vi "Custom Device Template Tool.vi"(4 "Extra Page Names (No Extension)":string[](array[string]), 6 "Open Project":bool=TRUE, 7 "Overwrite Existing (T)":bool=TRUE, 8 "error in (no error)":errorcluster, 9 "Execution Mode":T1, 10 "Custom Device Name (No Extension)":string, 11 "Target Folder":path=path "c:/temp") -> (0 "error out":errorcluster, 1 "Custom Device Library path":path, 2 "Custom Device Project path":path)   [LabVIEW 2020, in "Custom Device Template Tool.lvlib"]
uses:
  <vilib>/NI VeriStand/Custom Device Tools/Custom Device Template Tool/Custom Device Template Tool.lvlib
  <vilib>/NI VeriStand/Custom Device API/Custom Device Execution Mode.ctl
  NationalInstruments.VeriStand.Internal
  <vilib>/NI VeriStand/Custom Device API/Initialization VI Template.vit
  <vilib>/NI VeriStand/Custom Device API/Page Template.vit
  <vilib>/NI VeriStand/Custom Device API/Inline Custom Device Driver VI Template (HW Interface).vit
  <vilib>/NI VeriStand/Custom Device API/Inline Custom Device Driver VI Template (Model Interface).vit
  <vilib>/NI VeriStand/Custom Device API/Custom Device API.lvlib
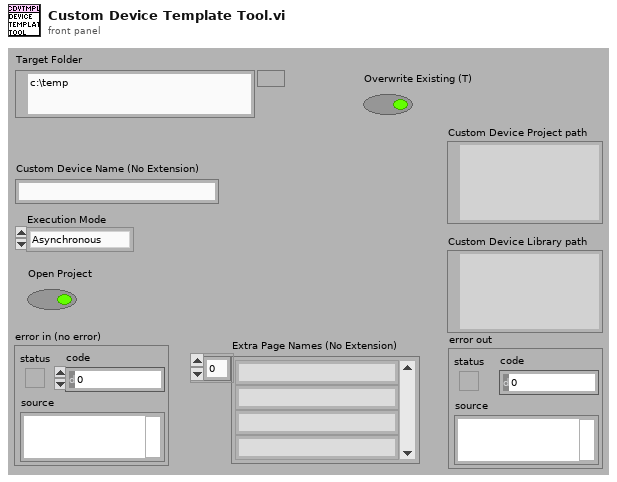
[diagram p1: front panel]
types:
  T1 = typedef "Custom Device API.lvlib/Custom Device Execution Mode.ctl" = enum16{"Asynchronous", "Inline HW Interface", "Inline Model Interface", "Inline Timing and Sync", "Asynchronous Timing and Sync"}
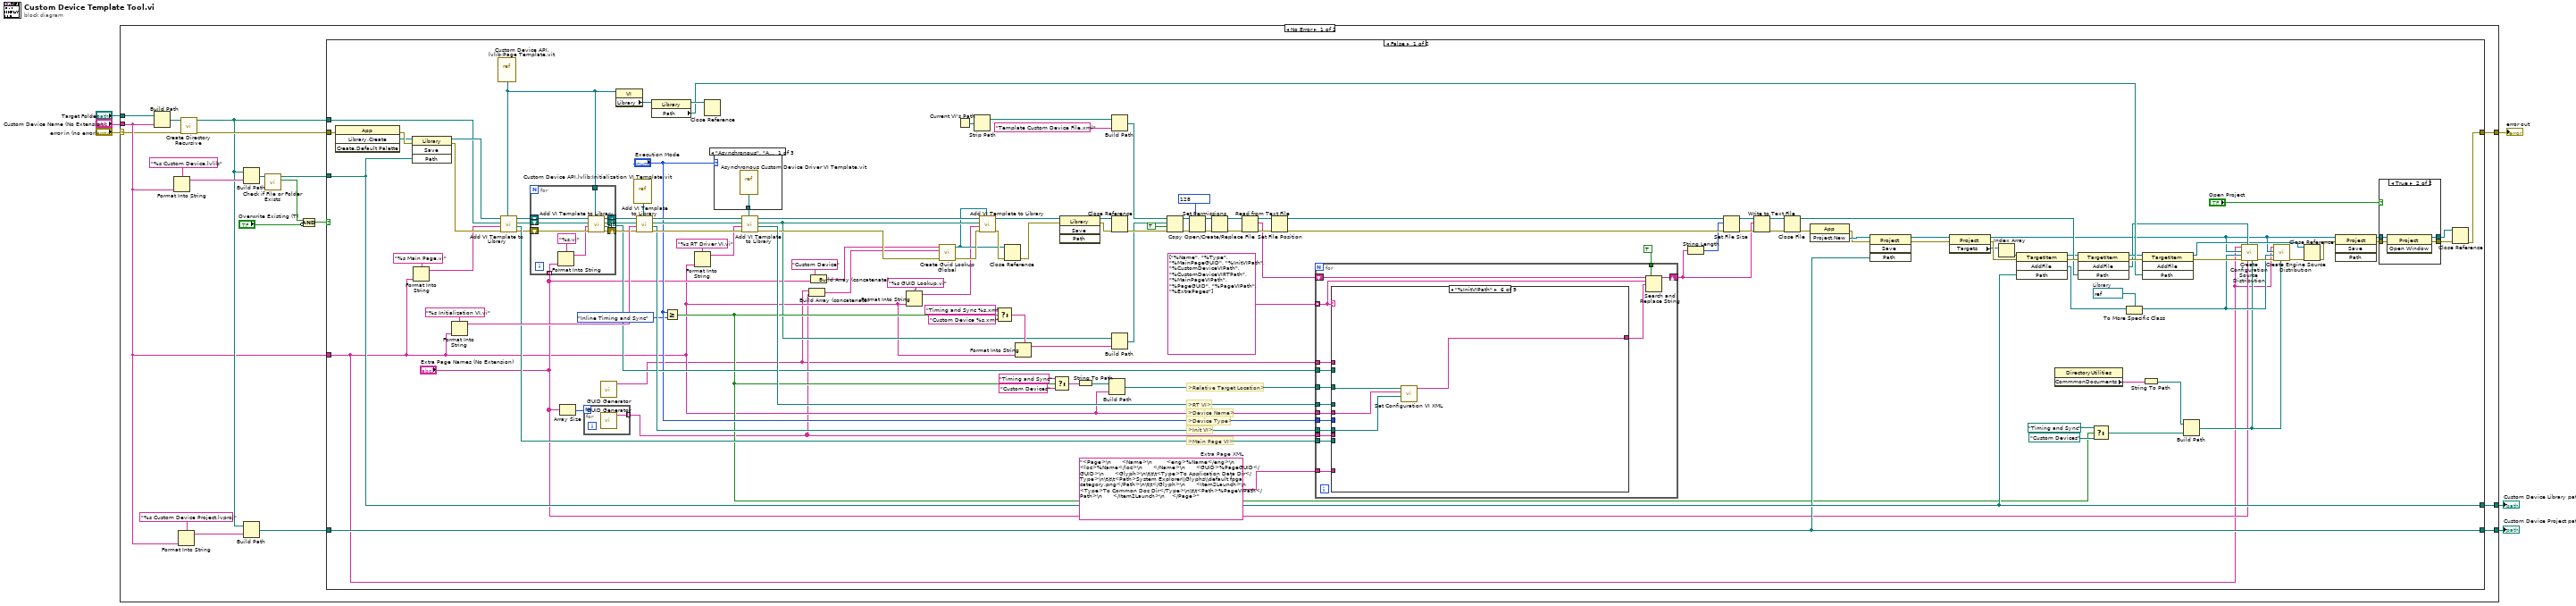
[diagram p0: block diagram]
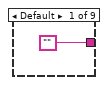
[diagram p3: hidden frame]
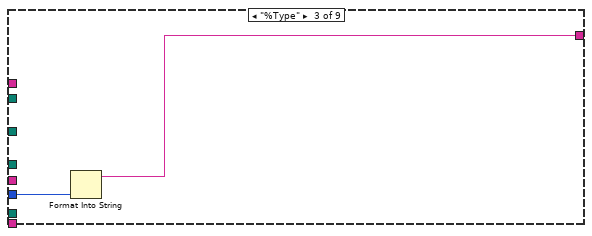
[diagram p5: hidden frame]
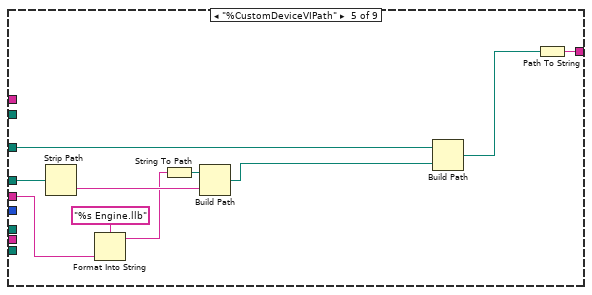
[diagram p7: hidden frame]
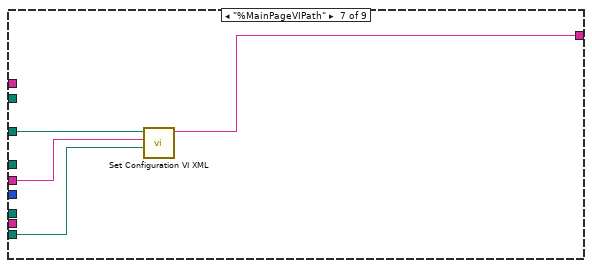
[diagram p8: hidden frame]
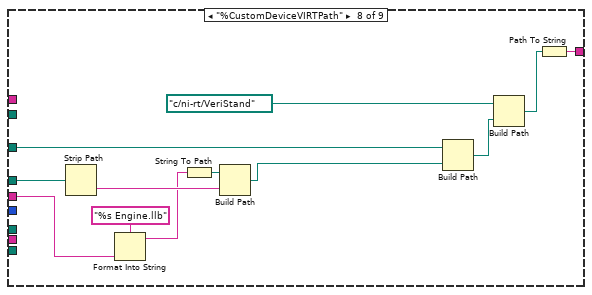
[diagram p9: hidden frame]
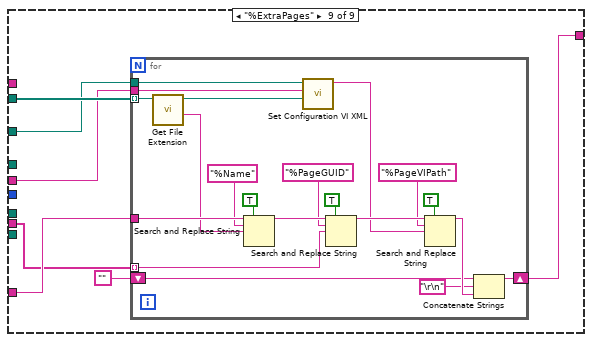
[diagram p10: hidden frame]
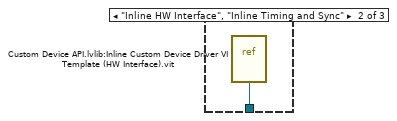
[diagram p11: hidden frame]
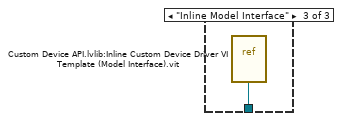
[diagram p12: hidden frame]
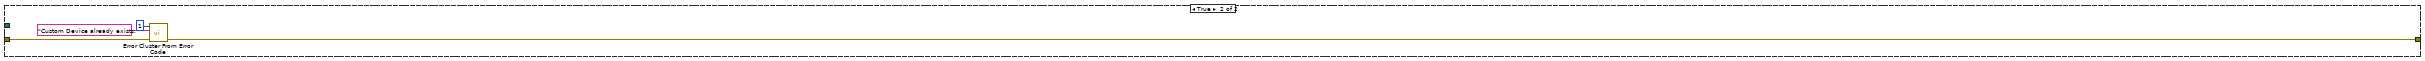
[diagram p13: hidden frame]
diagram:
  n1 = case shown="No Error" "error in (no error)" {
    selector: "error in (no error)" -> [w9 w256]
    tunnel: "Target Folder" -> [w21 _]
    tunnel: [w20 w256] -> w5
    tunnel: "Custom Device Name (No Extension)" -> [w16 _]
    tunnel: [w8 _] -> w2
    tunnel: [w7 _] -> w1
    frame No Error {
      n2 = Build Path(base path=w21, name or relative path=w16) -> (appended path=w25:path)
      n3 = Format Into String(format string="%s Custom Device.lvlib", w16) -> (resulting string=w22:string)  [unwired: 2 in, 1 out]
      n4 = Format Into String(format string="%s Custom Device Project.lvproj", w16) -> (resulting string=w19:string)  [unwired: 2 in, 1 out]
      n5 = call <vilib>:"Create Directory Recursive.vi"("error in (no error)"=w9, "directory"=w25) -> ("error out"=w23:errorcluster, "directory copy"=w17:path)  [unwired: 1 in, 3 out]
      n6 = Build Path(base path=w17, name or relative path=w22) -> (appended path=w14:path)
      n7 = Build Path(base path=w17, name or relative path=w19) -> (appended path=w15:path)
      n8 = call <vilib>:"Check if File or Folder Exists.vi"("path"=w14) -> ("file or folder exists?"=w12:bool, "dup path"=w13:path)  [unwired: 1 in, 8 out]
      n9 = Compound Arithmetic op=AND(w12, invert "Overwrite Existing (T)") -> (w10:bool)
      n10 = case shown="False" w10 {
        tunnel: w23 -> [w145 w255]
        tunnel: [w93 w254] -> w20
        tunnel: w17 -> [w84 _]
        tunnel: w16 -> [w31 _]
        tunnel: w15 -> [w57 _]
        tunnel: w13 -> [w58 _]
        tunnel: [w58 _] -> w8
        tunnel: [w57 _] -> w7
        frame False {
          w59 = "<Page>\n      <Name>\n        <eng>%Name</eng>\n        <loc>%Name</loc>\n      </Name>\n      <GUID>%PageGUID</GUID>\n      <Glyph>\n\t\t\t<Type>To Application Data Dir</Type>\n\t\t\t<Path>System Explorer\\Glyphs\\default fpga category.png</Path>\n\t\t</Glyph>\n      <Item2Launch>\n        <Type>To Common Doc Dir</Type>\n\t\t<Path>%PageVIPath</Path>\n      </Item2Launch>\n    </Page>"  # Extra Page XML
          w78 = refnum<vi> refnum  # Library
          # ">Relative Target Location>"
          # ">Device Type>"
          # ">Main Page VI>"
          # ">RT VI>"
          # ">Device Name>"
          # ">Init VI>"
          n11 = invoke class="App" method="Library.Create"(error in=w145) -> (error out=w147:errorcluster, "Create Library"=w146:refnum<vi>)  [unwired: 3 in, 2 out]
          n12 = invoke class="Library" method="Save"(reference=w146, error in=w147, "Path"=w58) -> (reference out=w143:refnum<vi>, error out=w148:errorcluster)  [unwired: 1 in, 2 out]
          n13 = Format Into String(format string="%s Main Page.vi", w31) -> (resulting string=w142:string)  [unwired: 2 in, 1 out]
          n14 = Format Into String(format string="%s Initialization VI.vi", w31) -> (resulting string=w139:string)  [unwired: 2 in, 1 out]
          n15 = vi-ref "Custom Device API.lvlib:Page Template.vit"() -> (w61:refnum<vi>)
          n16 = call <vilib>:"Add VI Template to Library.vi"("Template VI Refnum"=w61, "error in"=w148, "VI Name"=w142, "Custom Device Folder"=w84, "Custom Device Library in"=w143) -> ("error out"=w63:errorcluster, "VI Path out"=w117:path, "Custom Device Folder out"=w65:path, "Custom Device Library out"=w67:refnum<vi>)  [unwired: 3 out]
          n17 = for {
            shift-right: [w161] -> w66
            shift-left: w67 -> [w164]
            shift-right: [w160] -> w64
            shift-left: w65 -> [w163]
            shift-right: [w159] -> w62
            shift-left: w63 -> [w162]
            tunnel: w61 -> [w165]
            tunnel: "Extra Page Names (No Extension)" -> [w157] mode=indexing
            tunnel: [w155] -> w60 mode=indexing
            n18 = Format Into String(format string="%s.vi", w157) -> (resulting string=w156:string)  [unwired: 2 in, 1 out]
            n19 = call <vilib>:"Add VI Template to Library.vi"("Template VI Refnum"=w165, "error in"=w162, "VI Name"=w156, "Custom Device Folder"=w163, "Custom Device Library in"=w164) -> ("error out"=w159:errorcluster, "VI Path out"=w155:path, "Custom Device Folder out"=w160:path, "Custom Device Library out"=w161:refnum<vi>)  [unwired: 3 out]
          }
          n20 = Array Size(array="Extra Page Names (No Extension)") -> (size(s)=w43:i32)
          n21 = for {
            N: w43 -> [_]
            tunnel: [w154] -> w30 mode=indexing
            n22 = call <vilib>:"GUID Generator.vi"() -> ("GUID"=w154:string)  [unwired: 11 out]
          }
          n23 = call <vilib>:"GUID Generator.vi"() -> ("GUID"=w28:string)  [unwired: 11 out]
          n24 = property class="VI"(reference=w61) -> ("Library"=w92:refnum<vi>)  [unwired: 1 in, 2 out]
          n25 = vi-ref "Custom Device API.lvlib:Initialization VI Template.vit"() -> (w140:refnum<vi>)
          n26 = call <vilib>:"Add VI Template to Library.vi"("Template VI Refnum"=w140, "error in"=w62, "VI Name"=w139, "Custom Device Folder"=w64, "Custom Device Library in"=w66) -> ("error out"=w149:errorcluster, "VI Path out"=w116:path, "Custom Device Folder out"=w134:path, "Custom Device Library out"=w135:refnum<vi>)  [unwired: 3 out]
          n27 = property class="Library"(reference=w92) -> (reference out=w91:refnum<vi>, "Path"=w89:path)  [unwired: 1 in, 1 out]
          n28 = Greater Or Equal?(x="Execution Mode", y=Custom_Device_Execution_Mode."Inline Timing and Sync") -> (x >= y?=w47:bool)
          n29 = Format Into String(format string="%s RT Driver VI.vi", w31) -> (resulting string=w138:string)  [unwired: 2 in, 1 out]
          n30 = Close Reference(reference=w91) -> ()  [unwired: 1 in, 1 out]
          n31 = case shown="\"Asynchronous\", \"Asynchronous Timing and Sync\"" "Execution Mode" {
            tunnel: [w249 w250 w251] -> w137
            frame "Asynchronous", "Asynchronous Timing and Sync" {
              n32 = vi-ref <vilib>:"Asynchronous Custom Device Driver VI Template.vit"() -> (w249:refnum<vi>)
            }
            frame "Inline HW Interface", "Inline Timing and Sync" {
              n33 = vi-ref "Custom Device API.lvlib:Inline Custom Device Driver VI Template (HW Interface).vit"() -> (w250:refnum<vi>)
            }
            frame "Inline Model Interface" {
              n34 = vi-ref "Custom Device API.lvlib:Inline Custom Device Driver VI Template (Model Interface).vit"() -> (w251:refnum<vi>)
            }
          }
          n35 = call <vilib>:"Add VI Template to Library.vi"("Template VI Refnum"=w137, "error in"=w149, "VI Name"=w138, "Custom Device Folder"=w134, "Custom Device Library in"=w135) -> ("error out"=w40:errorcluster, "VI Path out"=w150:path, "Custom Device Folder out"=w38:path, "Custom Device Library out"=w41:refnum<vi>)  [unwired: 3 out]
          n36 = Build Array (concatenate)(w28, w30) -> (w29:string[])
          n37 = Build Array (concatenate)("Custom Device", "Extra Page Names (No Extension)") -> (w32:string[])
          n38 = Format Into String(format string="%s GUID Lookup.vi", w31) -> (resulting string=w35:string)  [unwired: 2 in, 1 out]
          n39 = call <vilib>:"Create Guid Lookup Global.vi"("error in (no error)"=w40, "GUIDs"=w29, "Page Names"=w32) -> ("error out"=w39:errorcluster, "Global VI Refnum"=w36:refnum<vi>)  [unwired: 7 in]
          n40 = Current VI's Path() -> (path=w83:path)
          n41 = Strip Path(path=w83) -> (stripped path=w82:path)  [unwired: 1 out]
          n42 = call <vilib>:"Add VI Template to Library.vi"("Template VI Refnum"=w36, "error in"=w39, "VI Name"=w35, "Custom Device Folder"=w38, "Custom Device Library in"=w41) -> ("error out"=w153:errorcluster, "Custom Device Library out"=w42:refnum<vi>)  [unwired: 5 out]
          n43 = Select(t="Timing and Sync %s.xml" ("format string"), s=w47, f="Custom Device %s.xml" ("format string")) -> (s? t:f=w52:string)
          n44 = Close Reference(reference=w36, error in (no error)=w153) -> (error out=w152:errorcluster)
          n45 = Format Into String(format string=w52, w31) -> (resulting string=w131:string)  [unwired: 2 in, 1 out]
          n46 = Select(t="Timing and Sync", s=w47, f="Custom Devices" ("name or relative path")) -> (s? t:f=w44:string)
          n47 = invoke class="Library" method="Save"(reference=w42, error in=w152) -> (reference out=w100:refnum<vi>, error out=w99:errorcluster)  [unwired: 2 in, 2 out]
          n48 = String To Path(string=w44) -> (path=w115:path)
          n49 = Build Path(base path=w115, name or relative path=w31) -> (appended path=w114:path)
          n50 = Build Path(base path=w82, name or relative path="Template Custom Device File.xml") -> (appended path=w132:path)
          n51 = Close Reference(reference=w100, error in (no error)=w99) -> (error out=w133:errorcluster)
          n52 = Build Path(base path=w38, name or relative path=w131) -> (appended path=w130:path)
          n53 = Copy(8:w133, 9:TRUE ("overwrite (F)"), 10:w130, 11:w132) -> (0:w127:errorcluster, 3:w128:path)  [unwired: 2 out]
          n54 = Set Permissions(7:i16 128 ("permissions"), 8:w127, 11:w128) -> (0:w125:errorcluster, 3:w126:path)  [unwired: 2 out]
          n55 = Open/Create/Replace File(file path (use dialog)=w126, error in=w125) -> (refnum out=w124:refnum<file>, error out=w123:errorcluster)  [unwired: 5 out]
          n56 = Read from Text File(file (use dialog)=w124, error in=w123) -> (refnum out=w122:refnum<file>, text=w119:string, error out=w121:errorcluster)  [unwired: 3 out]
          n57 = Set File Position(refnum=w122, error in=w121) -> (refnum out=w113:refnum<file>, error out=w112:errorcluster)  [unwired: 2 out]
          n58 = for {
            tunnel: string[] ["%Name", "%Type", "%MainPageGUID", "%InitVIPath", "%CustomDeviceVIPath", "%CustomDeviceVIRTPath", "%MainPageVIPath", "%PageGUID", "%PageVIPath", "%ExtraPages"] ("array") -> [w182] mode=indexing
            shift-right: [w176] -> w108
            shift-left: w119 -> [w186]
            tunnel: TRUE ("replace all? (F)") -> [w185]
            tunnel: w31 -> [w184]
            tunnel: "Execution Mode" -> [w181]
            tunnel: w117 -> [w180]
            tunnel: w116 -> [w179]
            tunnel: w150 -> [w178]
            tunnel: w114 -> [w177]
            tunnel: w60 -> [w175]
            tunnel: w59 -> [w174]
            tunnel: w30 -> [w173]
            tunnel: w28 -> [w172]
            n59 = case shown="\"%InitVIPath\"" w182 {
              tunnel: w184 -> [_ w188 _ _ w197 w203 w208 w212 w226]
              tunnel: ["" w188 w189 w191 w200 w202 w209 w217 w224] -> w183
              tunnel: w181 -> [_ _ w190 _ _ _ _ _ _]
              tunnel: w180 -> [_ _ _ _ _ _ w206 _ _]
              tunnel: w179 -> [_ _ _ _ _ w204 _ _ _]
              tunnel: w178 -> [_ _ _ _ w199 _ _ w213 _]
              tunnel: w177 -> [_ _ _ _ w192 w205 w207 w221 w227]
              tunnel: w175 -> [_ _ _ _ _ _ _ _ w228]
              tunnel: w174 -> [_ _ _ _ _ _ _ _ w223]
              tunnel: w173 -> [_ _ _ _ _ _ _ _ w222]
              tunnel: w172 -> [_ _ _ w191 _ _ _ _ _]
              frame Default {
              }
              frame "%Name" {
              }
              frame "%Type" {
                n60 = Format Into String(w190) -> (resulting string=w189:string)  [unwired: 3 in, 1 out]
              }
              frame "%MainPageGUID" {
              }
              frame "%CustomDeviceVIPath" {
                n61 = Strip Path(path=w199) -> (name=w201:string)  [unwired: 1 out]
                n62 = Format Into String(format string="%s Engine.llb", w197) -> (resulting string=w196:string)  [unwired: 2 in, 1 out]
                n63 = String To Path(string=w196) -> (path=w195:path)
                n64 = Build Path(base path=w195, name or relative path=w201) -> (appended path=w194:path)
                n65 = Build Path(base path=w192, name or relative path=w194) -> (appended path=w193:path)
                n66 = Path To String(path=w193) -> (string=w200:string)
              }
              frame "%InitVIPath" {
                n67 = call <vilib>:"Set Configuration VI XML.vi"("Configuration VI Path"=w204, "Custom Device Name (No Extension)"=w203, "Relative Target Location"=w205) -> ("XML String"=w202:string)  [unwired: 8 out]
              }
              frame "%MainPageVIPath" {
                n68 = call <vilib>:"Set Configuration VI XML.vi"("Configuration VI Path"=w206, "Custom Device Name (No Extension)"=w208, "Relative Target Location"=w207) -> ("XML String"=w209:string)  [unwired: 8 out]
              }
              frame "%CustomDeviceVIRTPath" {
                n69 = Strip Path(path=w213) -> (name=w216:string)  [unwired: 1 out]
                n70 = Format Into String(format string="%s Engine.llb", w212) -> (resulting string=w211:string)  [unwired: 2 in, 1 out]
                n71 = String To Path(string=w211) -> (path=w214:path)
                n72 = Build Path(base path=w214, name or relative path=w216) -> (appended path=w210:path)
                n73 = Build Path(base path=w221, name or relative path=w210) -> (appended path=w219:path)
                n74 = Build Path(base path=path "c:/ni-rt/VeriStand" ("appended path"), name or relative path=w219) -> (appended path=w218:path)
                n75 = Path To String(path=w218) -> (string=w217:string)
              }
              frame "%ExtraPages" {
                n76 = for {
                  tunnel: w228 -> [w248] mode=indexing
                  tunnel: w227 -> [w236]
                  tunnel: w226 -> [w235]
                  tunnel: w223 -> [w247]
                  shift-right: [w232] -> w224
                  shift-left: "" -> [w231]
                  tunnel: w222 -> [w229] mode=indexing
                  n77 = call <vilib>:"Get File Extension.vi"("file"=w248) -> ("filename without extension"=w245:string, "dup file"=w237:path)  [unwired: 1 in, 8 out]
                  n78 = Search and Replace String(replace all?=TRUE ("replace all? (F)"), input string=w247, search string="%Name", replace string=w245) -> (result string=w242:string)  [unwired: 1 in, 6 out]
                  n79 = call <vilib>:"Set Configuration VI XML.vi"("Configuration VI Path"=w237, "Custom Device Name (No Extension)"=w235, "Relative Target Location"=w236) -> ("XML String"=w234:string)  [unwired: 8 out]
                  n80 = Search and Replace String(replace all?=TRUE ("replace all? (F)"), input string=w242, search string="%PageGUID", replace string=w229) -> (result string=w239:string)  [unwired: 1 in, 6 out]
                  n81 = Search and Replace String(replace all?=TRUE ("replace all? (F)"), input string=w239, search string="%PageVIPath", replace string=w234) -> (result string=w233:string)  [unwired: 1 in, 6 out]
                  n82 = Concatenate Strings(w231, "\r\n", w233) -> (w232:string)
                }
              }
            }
            n83 = Search and Replace String(replace all?=w185, input string=w186, search string=w182, replace string=w183) -> (result string=w176:string)  [unwired: 1 in, 6 out]
          }
          n84 = String Length(string=w108) -> (length=w111:i32)
          n85 = Set File Size(4:w112, 6:w111, 7:w113) -> (0:w109:errorcluster, 3:w110:refnum<file>)
          n86 = Write to Text File(file (use dialog)=w110, text=w108, error in=w109) -> (refnum out=w106:refnum<file>, error out=w107:errorcluster)  [unwired: 2 out]
          n87 = Close File(refnum=w106, error in=w107) -> (path=w97:path, error out=w103:errorcluster)
          n88 = invoke class="App" method="Project.New"(error in=w103) -> (error out=w70:errorcluster, "Project:New"=w71:refnum<vi>)  [unwired: 2 in, 1 out]
          n89 = invoke class="Project" method="Save"(reference=w71, error in=w70, "Path"=w57) -> (reference out=w69:refnum<vi>, error out=w68:errorcluster)  [unwired: 1 in, 2 out]
          n90 = property class="Project"(reference=w69, error in=w68) -> (reference out=w74:refnum<vi>, error out=w151:errorcluster, "Targets"=w102:refnum<vi>[])
          n91 = Index Array(array=w102) -> (element=w101:refnum<vi>)  [unwired: 1 in]
          n92 = invoke class="TargetItem" method="AddFile"(reference=w101, error in=w151, "Path"=w58) -> (reference out=w88:refnum<vi>, error out=w98:errorcluster, "AddFile"=w79:refnum<vi>)  [unwired: 1 in, 1 out]
          n93 = property class="DirectoryUtilities"() -> ("CommmonDocuments"=w27:string)  [unwired: 2 in, 2 out]
          n94 = invoke class="TargetItem" method="AddFile"(reference=w88, error in=w98, "Path"=w97) -> (reference out=w87:refnum<vi>, error out=w90:errorcluster, "AddFile"=w80:refnum<vi>)  [unwired: 1 in, 1 out]
          n95 = Select(t=path "Timing and Sync" ("App All User Path"), s=w47, f=path "Custom Devices" ("App All User Path")) -> (s? t:f=w48:path)
          n96 = To More Specific Class(target class=w78, reference=w79) -> (specific class reference=w73:refnum<vi>)  [unwired: 1 in, 1 out]
          n97 = invoke class="TargetItem" method="AddFile"(reference=w87, error in=w90, "Path"=w89) -> (reference out=w77:refnum<vi>, error out=w81:errorcluster)  [unwired: 1 in, 2 out]
          n98 = String To Path(string=w27) -> (path=w26:path)
          n99 = Build Path(base path=w26, name or relative path=w48) -> (appended path=w51:path)
          n100 = call <vilib>:"Create Configuration Source Distribution.vi"("Base Path"=w51, "Extra Page Names"="Extra Page Names (No Extension)", "XML File Refnum"=w80, "error in (no error)"=w81, "Library Refnum"=w73, "Project Refnum"=w74, "Custom Device Name"=w31) -> ("error out"=w75:errorcluster)  [unwired: 4 out]
          n101 = call <vilib>:"Create Engine Source Distribution.vi"("Base Path"=w51, "error in (no error)"=w75, "Library Refnum"=w73, "Project Refnum"=w74, "Custom Device Name"=w31) -> ("error out"=w72:errorcluster)  [unwired: 6 out]
          n102 = Close Reference(reference=w77, error in (no error)=w72) -> (error out=w76:errorcluster)
          n103 = invoke class="Project" method="Save"(reference=w74, error in=w76) -> (reference out=w86:refnum<vi>, error out=w85:errorcluster)  [unwired: 2 in, 2 out]
          n104 = case shown="True" "Open Project" {
            tunnel: w85 -> [w167 w171]
            tunnel: w86 -> [w166 w170]
            tunnel: [w167 w169] -> w95
            tunnel: [w166 w168] -> w94
            frame False {
            }
            frame True {
              n105 = invoke class="Project" method="Open Window"(reference=w170, error in=w171) -> (reference out=w168:refnum<vi>, error out=w169:errorcluster)  [unwired: 1 in, 1 out]
            }
          }
          n106 = Close Reference(reference=w94, error in (no error)=w95) -> (error out=w93:errorcluster)
        }
        frame True {
          n107 = call <vilib>:"Error Cluster From Error Code.vi"("error in (no error)"=w255, "error message (\"\")"="Custom Device already exists." ("error message (\"\")"), "error code (0)"=1) -> ("error out"=w254:errorcluster)  [unwired: 1 in, 5 out]
        }
      }
    }
    frame Error {
    }
  }
  "error out" <- w5
  "Custom Device Library path" <- w2
  "Custom Device Project path" <- w1
